vi "Main_v2.vi"() -> ()   [LabVIEW 2023]
doc: "Develop by: B.S. Brandon Obregón Garita \n\nRequirements of the project: \n- Read Analog Data from Current and Voltage Sensor with NI-6000\n- Measure frequency of wind turbine with optocuopler sensor. \n\nExplain of the code: \n- Due to necessity of measure from 2 different types of sensor (analog and digital), we implement a philosophy of Producer / Consumer Loops. \n- Firstly, DAQ ports are initialize with their respective settings, after that, the queues are created. \n- We split the measures: the reading of analog data executes in parallel with the reading of digital data. \n- For other hand, when the data is save on the buffer (queue) the software read them, processing occurs and data is deleted from buffer. \n- If the user needs save data a botton is present in the front panel, when de boolean is true will request a name of the file (notece that file path is already selected) and the process of saving will begin. \n- Data is save into a .csv file and it could be process with Python, Excel, Minitab, Matlab etc. \n- When the user press stop all instance will finish and the program will stop successfully. \n\nSoftware repocitory:\n https://github.com/BrandonOG13/DAQTURBINE"
uses:
  Selector.ctl
  <vilib>/DAQmx/read.llb/DAQmx Read (Analog 2D DBL NChan NSamp).vi
  <vilib>/DAQmx/read.llb/DAQmx Read (Digital Bool 1Line 1Point).vi
  <vilib>/DAQmx/miscellaneous.llb/DAQmx Fill In Error Info.vi
  Proyecto/Test_Libraries.lvlib
panel:
  out "Refresh time (s)":dbl
  in  "Number of samples":i32=50
  in  "Rate (Hz)":dbl=100.0
  out "Path":bool
  out "RPM":bool
  out "Voltmeter":bool
  out "ACS712":bool
  in  "Data Acquisition":bool
  in  "File Path":path
  in  "Time":i32=60
  out "Iteration":i32
  in  "Main":T1(tab)
  out "Voltage":dbl(graph)
  out "Current":dbl(graph)
  out "Power":dbl(graph)
  out "Velocity":dbl(graph)
  in  "Stop":bool
  out "Current [A]":dbl(knob) scale=0.0..10.0 scale format="%#_3g"
  out "Voltage [V]":dbl(knob) scale=0.0..10.0
  out "Power [W]":dbl(knob) scale=0.0..500.0
  out "Velocity [RPM]":dbl(knob) scale=0.0..1800.0
  out "Stop 2":bool
  # "TEST BENCH FOR WIND TURBINE"
  # "Status & Error"
  # "DAQ Settings"
  # "Save data"
  # "Instituto Tecnológico de Costa Rica"
  # "Laboratorio de Investigación en Energía Eólica"
  # "Developer: B.S. Student. Brandon Obregón Garita"
  # "Email: bobregon@estudiantec.cr"
  # "Version: 1.0"
  # "Last modification: 28/08/2023"
  # "Optocoupler channel: Digital sensor, operational voltage: 5 [V].\n\nOut connected to PFI 0. GND connected to D.GND. \nVCC required 5 V of  external device [DC Power Supply]"
  # "Common ground for analog sensors"
  # "Current Channel [ACS712 - 30A]: Sensor required 5V of an external device. \nSensibility [based on Lab Test]: 0.070 mV/A\nOut connected to AI 0. GND connected to common ground\nMax Current: 30 A."
  # "Voltage Channel: Measured from voltage divider, protected by Zener Diode. Max Volt: 4.7 [V]\nPositive connected to AI 1 | Negative connected to common ground\nVoltage divider: 10kOhm & 1kOhm | Gain: Vturbine = 11*Vmeasured"
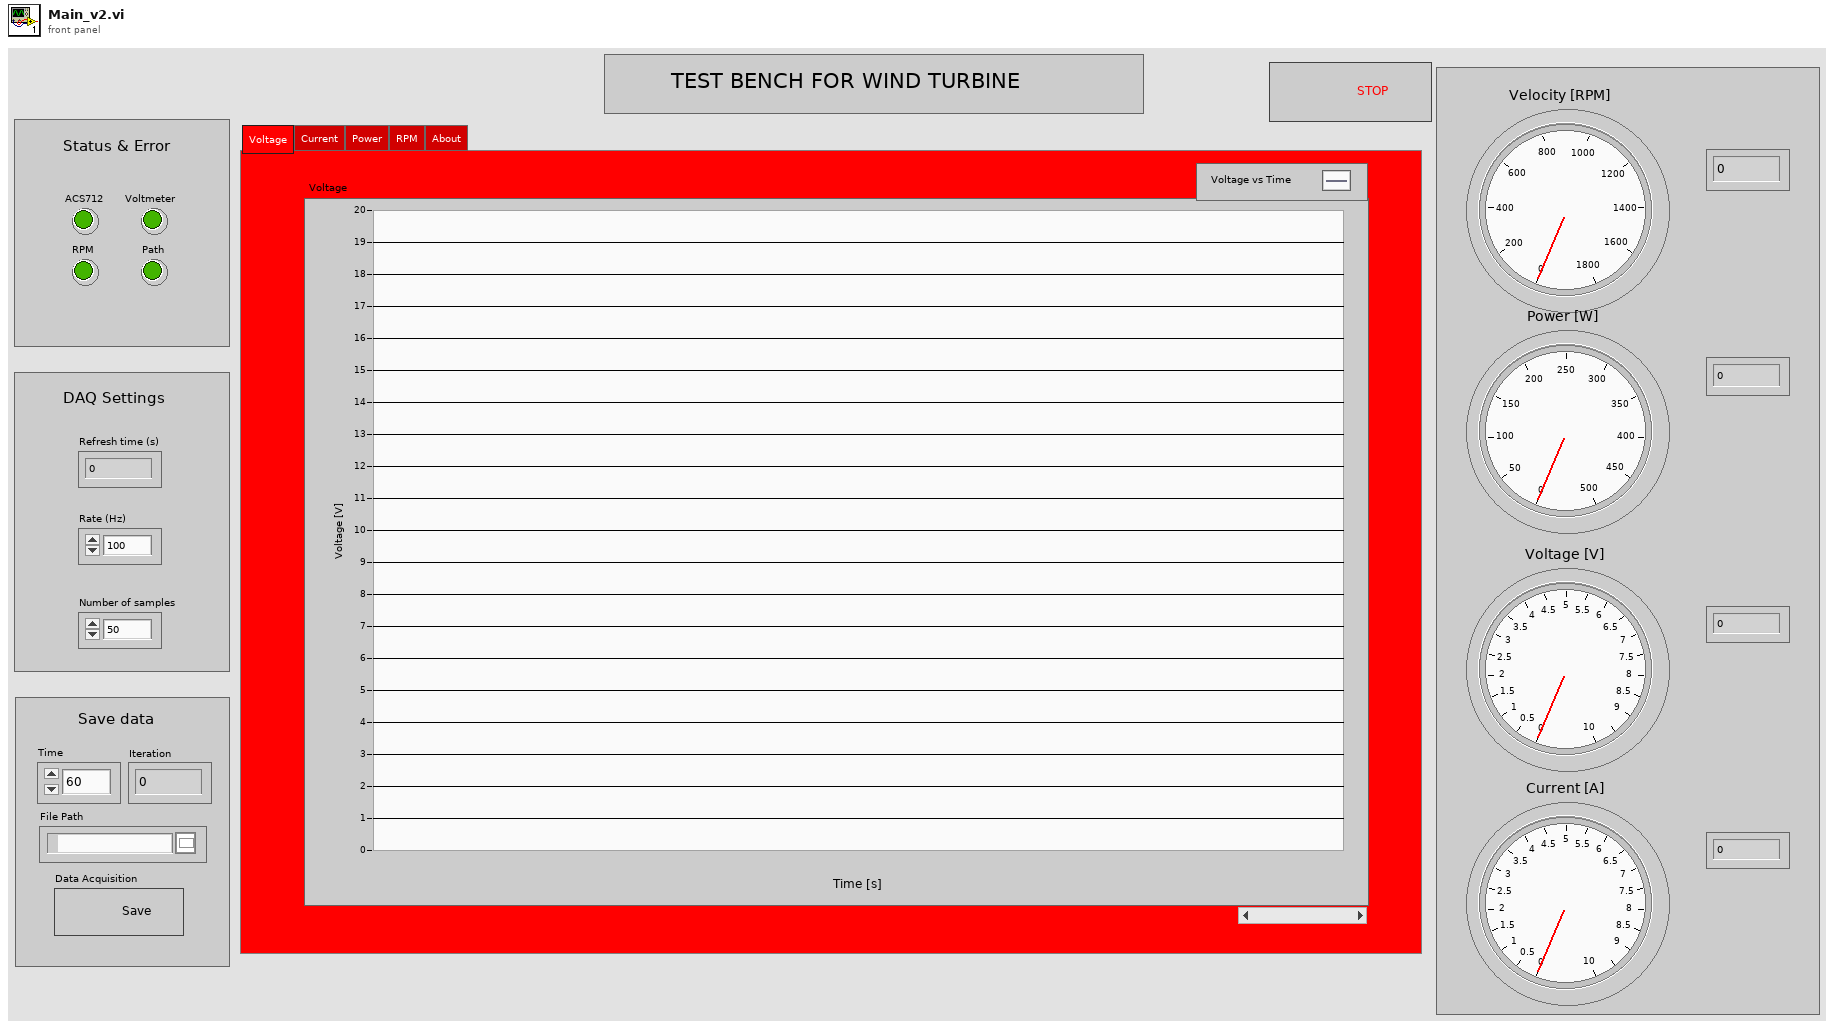
[diagram p1: front panel]
types:
  T1 = enum32{"Voltage", "Current", "Power", "RPM", "About"}
  T2 = typedef "Test_Libraries.lvlib/Selector.ctl" = enum16{"Stand By", "Path", "Measurement", "End"}
  T3 = cluster{"[0]":dbl, "[1]":dbl, "[2]":dbl, "[3]":dbl, "[4]":dbl, "[5]":dbl, "[6]":dbl, "[7]":dbl, "[8]":dbl}
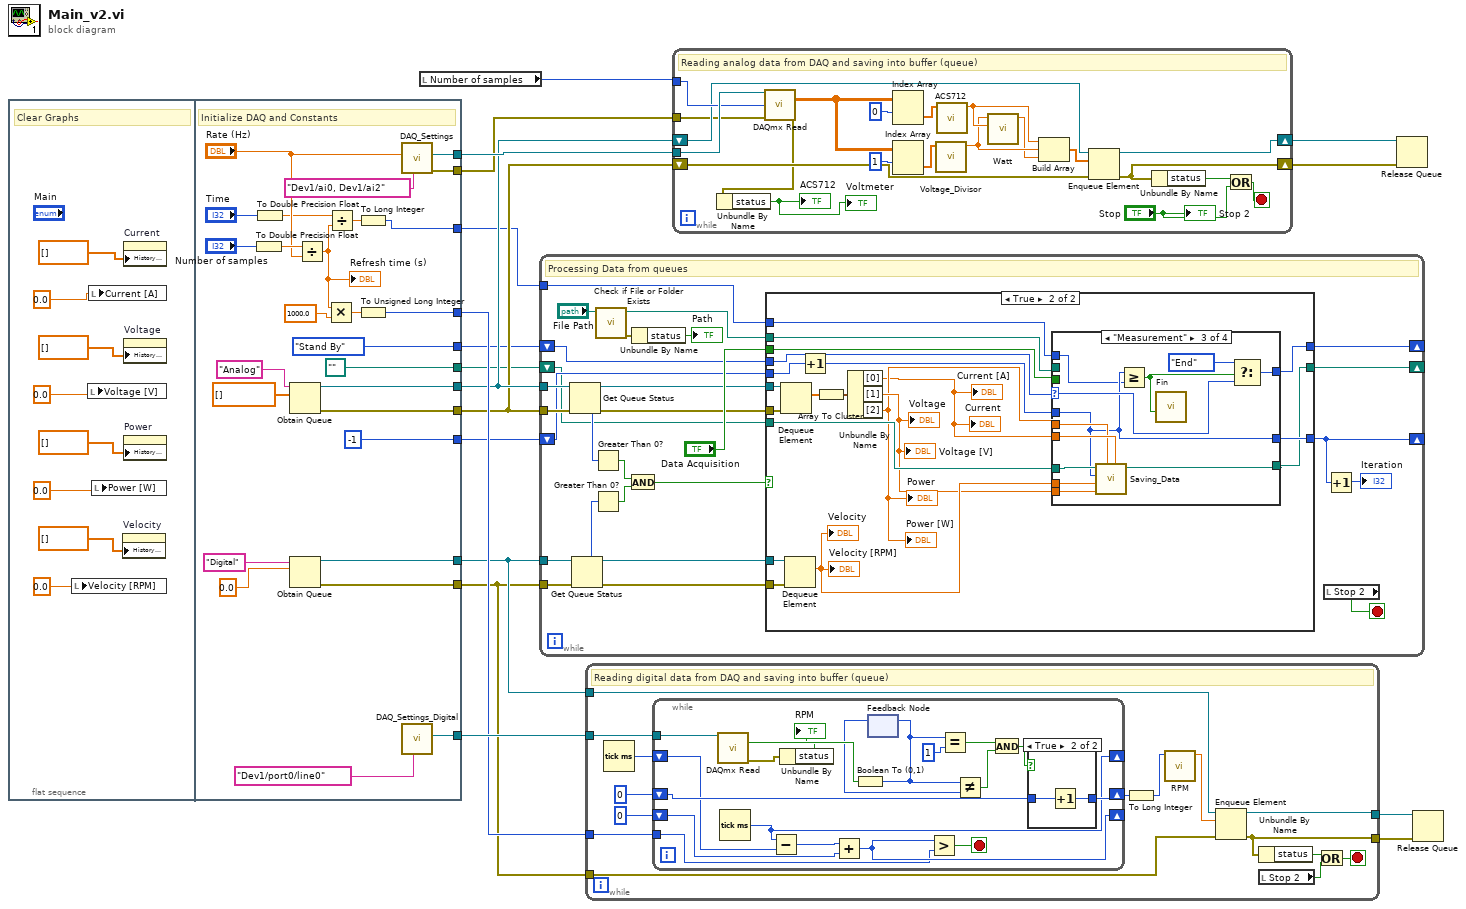
[diagram p0: block diagram]
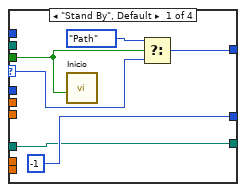
[diagram p3: hidden frame]
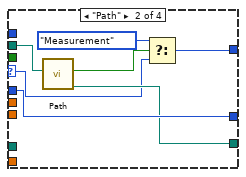
[diagram p4: hidden frame]
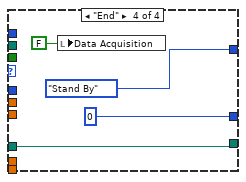
[diagram p5: hidden frame]
diagram:
  n1 = flat-sequence {
    tunnel: [w48] -> w14
    tunnel: [w47] -> w17
    tunnel: [w46] -> w3
    tunnel: [w44] -> w9
    tunnel: [w43] -> w10
    tunnel: [w42] -> w8
    tunnel: [w41] -> w7
    tunnel: [w37] -> w13
    tunnel: [Selector."Stand By" ("Enum")] -> w5
    tunnel: [path "" ("appended path")] -> w4
    tunnel: [-1] -> w2
    tunnel: [w26] -> w1
    frame #0 {
      # "Clear Graphs"
      n2 = local write "Velocity [RPM]"(0.0 ("Velocity [RPM]")) -> ()
      n3 = local write "Voltage [V]"(0.0 ("Voltage [V]")) -> ()
      n4 = local write "Current [A]"(0.0 ("Current [A]")) -> ()
      n5 = local write "Power [W]"(0.0 ("Power [W]")) -> ()
      n6 = property on="Velocity" class="WFChart (strict)"("History Data"=dbl[] []) -> ()  [unwired: 2 in, 2 out]
      n7 = property on="Current" class="WFChart (strict)"("History Data"=dbl[] []) -> ()  [unwired: 2 in, 2 out]
      n8 = property on="Voltage" class="WFChart (strict)"("History Data"=dbl[] []) -> ()  [unwired: 2 in, 2 out]
      n9 = property on="Power" class="WFChart (strict)"("History Data"=dbl[] []) -> ()  [unwired: 2 in, 2 out]
    }
    frame #1 {
      # "Initialize DAQ and Constants"
      n10 = To Double Precision Float(number="Number of samples") -> (double precision float=w45:dbl)
      n11 = To Double Precision Float(number="Time") -> (double precision float=w30:dbl)
      n12 = Obtain Queue(name (unnamed)="Analog", element data type=dbl[] []) -> (queue out=w43:refnum<queue>, error out=w44:errorcluster)  [unwired: 3 in, 1 out]
      n13 = Obtain Queue(name (unnamed)="Digital", element data type=0.0) -> (queue out=w42:refnum<queue>, error out=w41:errorcluster)  [unwired: 3 in, 1 out]
      n14 = Divide(x=w45, y="Rate (Hz)") -> (x/y=w29:dbl)
      "Refresh time (s)" <- w29
      n15 = Multiply(x=w29, y=1000.0) -> (x*y=w38:dbl)
      n16 = Divide(x=w30, y=w29) -> (x/y=w28:dbl)
      n17 = To Long Integer(number=w28) -> (32bit integer=w46:i32)
      n18 = To Unsigned Long Integer(number=w38) -> (unsigned 32bit integer=w37:u32)
      n19 = call "DAQ_Settings.vi"("Channel"=tag "Dev1/ai0, Dev1/ai2" ("physical channels"), "rate"="Rate (Hz)") -> ("error out"=w26:errorcluster, "task out"=w47:refnum<k21>)  [unwired: 8 in]
      n20 = call "DAQ_Settings_Digital.vi"("lines"=tag "Dev1/port0/line0") -> ("task out"=w48:refnum<k21>)  [unwired: 9 in, 1 out]
    }
  }
  n21 = local read "Number of samples"() -> (w6:i32)
  n22 = while {
    tunnel: w10 -> [w78]
    tunnel: w9 -> [w77]
    tunnel: w8 -> [w75]
    tunnel: w7 -> [w74]
    shift-right: [w58] -> _
    shift-left: w5 -> [w62]
    shift-right: [w57] -> _
    shift-left: w4 -> [w60]
    tunnel: w3 -> [w61]
    shift-right: [w54] -> _
    shift-left: w2 -> [w63]
    stop <- w65 stop-if-true
    # "Processing Data from queues"
    n23 = Get Queue Status(queue=w78, error in (no error)=w77) -> (queue out=w69:refnum<queue>, error out=w68:errorcluster, # elements in queue=w76:i32)  [unwired: 1 in, 5 out]
    n24 = Get Queue Status(queue=w75, error in (no error)=w74) -> (queue out=w67:refnum<queue>, error out=w66:errorcluster, # elements in queue=w73:i32)  [unwired: 1 in, 5 out]
    n25 = Greater Than 0?(x=w76) -> (x > 0?=w72:bool)
    n26 = Greater Than 0?(x=w73) -> (x > 0?=w71:bool)
    n27 = call <vilib>:"Check if File or Folder Exists.vi"("path"="File Path") -> ("error out"=w56:errorcluster, "dup path"=w59:path)  [unwired: 8 in, 1 out]
    n28 = And(x=w72, y=w71) -> (x .and. y?=w70:bool)
    n29 = Unbundle By Name(w56) -> ("status"=→"Path":bool)
    n30 = case shown="True" w70 {
      tunnel: w69 -> [_ w101]
      tunnel: w68 -> [_ w100]
      tunnel: w67 -> [_ w99]
      tunnel: w66 -> [_ w98]
      tunnel: w63 -> [w80 w91]
      tunnel: w62 -> [w82 w90]
      tunnel: "Data Acquisition" -> [_ w88]
      tunnel: w61 -> [_ w87]
      tunnel: w60 -> [w81 w102]
      tunnel: w59 -> [_ w86]
      tunnel: [w80 w85] -> w54
      tunnel: [w82 w84] -> w58
      tunnel: [w81 w83] -> w57
      frame False {
      }
      frame True {
        n31 = Dequeue Element(queue=w101, error in (no error)=w100) -> (element=w97:dbl[])  [unwired: 1 in, 3 out]
        n32 = Dequeue Element(queue=w99, error in (no error)=w98) -> (element=w95:dbl)  [unwired: 1 in, 3 out]
        "Velocity" <- w95
        "Velocity [RPM]" <- w95
        n33 = Increment(x=w91) -> (x+1=w89:i32)
        n34 = Array To Cluster(array=w97) -> (cluster=w96:T3)
        n35 = Unbundle By Name(w96) -> ("[0]"=w92:dbl, "[1]"=w94:dbl, "[2]"=w93:dbl)
        "Current" <- w92
        "Current [A]" <- w92
        "Voltage" <- w94
        "Voltage [V]" <- w94
        "Power" <- w93
        "Power [W]" <- w93
        n36 = case shown="\"Measurement\"" w90 {
          selector: w90 -> [w106 w111 w125 _]
          tunnel: w92 -> [_ _ w121 _]
          tunnel: w93 -> [_ _ w120 _]
          tunnel: w94 -> [_ _ w119 _]
          tunnel: w95 -> [_ _ w117 _]
          tunnel: w89 -> [_ w115 w118 _]
          tunnel: [-1 ("Count+1") w115 w118 0 ("Iteración")] -> w85
          tunnel: w88 -> [w103 _ _ _]
          tunnel: [w105 w112 w123 Selector."Stand By" ("Enum")] -> w84
          tunnel: w87 -> [_ _ w116 _]
          tunnel: [w104 w114 w126 w128] -> w83
          tunnel: w102 -> [w104 _ w126 w128]
          tunnel: w86 -> [_ w109 _ _]
          frame "Stand By", Default {
            n37 = call "Inicio"("Enable"=w103) -> ()  [unwired: 9 in, 2 out]
            n38 = Select(t=Selector."Path" ("Enum"), s=w103, f=w106) -> (s? t:f=w105:T2)
          }
          frame "Path" {
            n39 = call "Path.vi"("selected path"=w109) -> ("appended path"=w114:path, "Boolean"=w110:bool)  [unwired: 7 in, 2 out]
            n40 = Select(t=Selector."Measurement" ("Enum"), s=w110, f=w111) -> (s? t:f=w112:T2)
          }
          frame "Measurement" {
            n41 = call "Saving_Data.vi"("Current"=w121, "Watt"=w120, "Voltage"=w119, "RPM"=w117, "Iteration"=w118, "file path"=w126) -> ()  [unwired: 6 in]
            n42 = Greater Or Equal?(x=w118, y=w116) -> (x >= y?=w122:bool)
            n43 = call "Fin"("Enable"=w122) -> ()  [unwired: 9 in, 2 out]
            n44 = Select(t=Selector."End" ("Enum"), s=w122, f=w125) -> (s? t:f=w123:T2)
          }
          frame "End" {
            n45 = local write "Data Acquisition"(FALSE ("Toma de datos")) -> ()
          }
        }
      }
    }
    n46 = local read "Stop 2"() -> (w65:bool)
    n47 = Increment(x=w54) -> (x+1=→"Iteration":i32)
  }
  n48 = while {
    tunnel: w8 -> [w144]
    tunnel: w7 -> [w143]
    tunnel: w14 -> [w145]
    tunnel: w13 -> [w137]
    tunnel: [w136] -> w12
    tunnel: [w134] -> w11
    stop <- w141 stop-if-true
    # "Reading digital data from DAQ and saving into buffer (queue)"
    n49 = Tick Count (ms)() -> (millisecond timer value=w139:u32)
    n50 = while {
      tunnel: w145 -> [w164]
      shift-right: [w157] -> w132
      shift-left: 0 -> [w158]
      shift-right: [w156] -> _
      shift-left: w139 -> [w155]
      shift-right: [w152] -> _
      shift-left: u32 0 -> [w153]
      tunnel: w137 -> [w148]
      stop <- w151 stop-if-true
      n51 = call-poly <vilib>:"DAQmx Read.vi"("task/channels in"=w164) -> ("data"=w163:bool, "error out"=w147:errorcluster)  [unwired: 12 in, 1 out]
      n52 = Tick Count (ms)() -> (millisecond timer value=w156:u32)
      n53 = Subtract(x=w156, y=w155) -> (x-y=w154:u32)
      n54 = Unbundle By Name(w147) -> ("status"=→"RPM":bool)
      n55 = Add(x=w154, y=w153) -> (x+y=w152:u32)
      n56 = Boolean To (0,1)(Boolean=w163) -> (0, 1=w150:i16)
      n57 = feedback-in #1(w150) -> ()
      n58 = feedback #1() -> (w149:i16)  [unwired: 1 in]
      n59 = Greater?(x=w152, y=w148) -> (0:w151:bool)
      n60 = Equal?(x=w150, y=i16 1) -> (x = y?=w161:bool)
      n61 = Not Equal?(x=w150, y=w149) -> (x != y?=w160:bool)
      n62 = And(x=w161, y=w160) -> (x .and. y?=w159:bool)
      n63 = case shown="True" w159 {
        tunnel: w158 -> [w165 w166]
        tunnel: [w165 w167] -> w157
        frame False {
        }
        frame True {
          n64 = Increment(x=w166) -> (x+1=w167:i32)
        }
      }
    }
    n65 = To Long Integer(number=w132) -> (32bit integer=w133:i32)
    n66 = call "RPM.vi"("Input"=w133) -> ("RPM"=w131:dbl)  [unwired: 10 in]
    n67 = Enqueue Element(queue=w144, element=w131, error in (no error)=w143) -> (queue out=w136:refnum<queue>, error out=w134:errorcluster)  [unwired: 1 in, 1 out]
    n68 = Unbundle By Name(w134) -> ("status"=w142:bool)
    n69 = local read "Stop 2"() -> (w135:bool)
    n70 = Or(x=w142, y=w135) -> (x .or. y?=w141:bool)
  }
  n71 = while {
    tunnel: w17 -> [w188]
    tunnel: w6 -> [w187]
    shift-right: [w178] -> w16
    shift-left: w10 -> [w181]
    shift-right: [w177] -> w15
    shift-left: w9 -> [w180]
    tunnel: w1 -> [w170]
    stop <- w175 stop-if-true
    # "Reading analog data from DAQ and saving into buffer (queue)"
    n72 = call-poly <vilib>:"DAQmx Read.vi"("task/channels in"=w188, "number of samples per channel"=w187, "error in"=w170) -> ("data"=w182:dbl[][], "error out"=w169:errorcluster)  [unwired: 10 in, 1 out]
    n73 = Unbundle By Name(w169) -> ("status"=→"ACS712" →"Voltmeter":bool)
    n74 = Index Array(array=w182, index (row)=0) -> (element=w184:dbl[])  [unwired: 1 in]
    n75 = Index Array(array=w182, index (row)=1) -> (element=w183:dbl[])  [unwired: 1 in]
    n76 = call "Voltage_Divisor.vi"("Voltage"=w183) -> ("Voltage_in"=w173:dbl)  [unwired: 10 in]
    n77 = call "ACS712.vi"("ACS712"=w184) -> ("Current"=w174:dbl)  [unwired: 10 in]
    n78 = call "Watt.vi"("Current"=w174, "Voltage_in"=w173) -> ("Watt"=w172:dbl)  [unwired: 9 in]
    n79 = Build Array(w174, w173, w172) -> (w179:dbl[])
    n80 = Enqueue Element(queue=w181, element=w179, error in (no error)=w180) -> (queue out=w178:refnum<queue>, error out=w177:errorcluster)  [unwired: 1 in, 1 out]
    n81 = Unbundle By Name(w177) -> ("status"=w176:bool)
    n82 = Or(x=w176, y="Stop") -> (x .or. y?=w175:bool)
    "Stop 2" <- "Stop"
  }
  n83 = Release Queue(queue=w16, error in (no error)=w15) -> ()  [unwired: 1 in, 3 out]
  n84 = Release Queue(queue=w12, error in (no error)=w11) -> ()  [unwired: 1 in, 3 out]
